vi "Read Area.vi"(8 "error in (no error)":errorcluster, 11 "Figure in":refnum<class "Figure.lvclass">) -> (0 "error out":errorcluster, 2 "Area":dbl, 3 "Figure out":refnum<class "Figure.lvclass">)   [LabVIEW 2021, in "Figure.lvclass"]
uses:
  Figure.lvclass
  Figure.lvclass/Figure.ctl
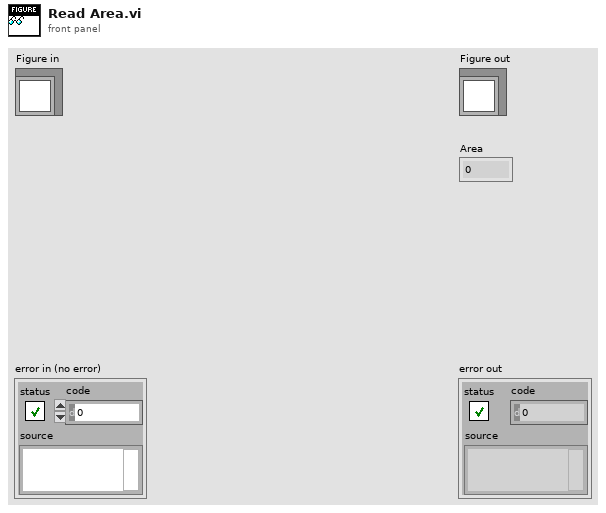
[diagram p1: front panel]
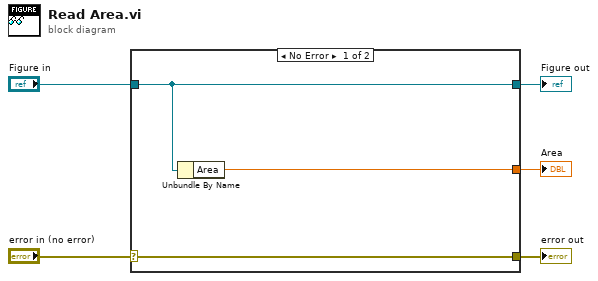
[diagram p0: block diagram]
diagram:
  n1 = case shown="No Error" "error in (no error)" {
    selector: "error in (no error)" -> [w8 w9]
    tunnel: [w8 w9] -> w4
    tunnel: [w7 w10] -> w2
    tunnel: "Figure in" -> [w7 w10]
    tunnel: [w6 _] -> w1
    frame No Error {
      n2 = Unbundle By Name(w7) -> ("Area"=w6:dbl)
    }
    frame Error {
    }
  }
  "error out" <- w4
  "Figure out" <- w2
  "Area" <- w1
